vi "Progress Bar Example with Multiple Instances.vi"() -> ()   [LabVIEW 2015]
uses:
  Library/New Job Status.vi
  Library/New Item Status.vi
  Library/Class/Finish.vi
  Library/Class/Bar.lvclass
  Library/Simple Progress Bar.lvlib
panel:
  out "Action in Progress 2":bool=TRUE
  out "Action in Progress":bool=TRUE
  out "error out 2":errorcluster
  in  "Step Duration mSec 2":u32=100
  in  "Steps 2":i32=150
  in  "Step Duration mSec":u32=1000
  in  "Steps":i32=10
  out "error out":errorcluster
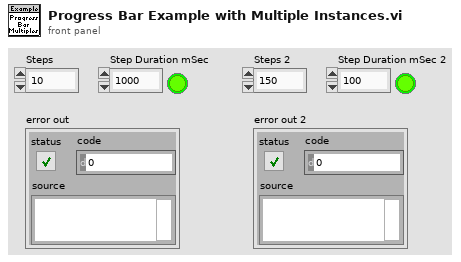
[diagram p1: front panel]
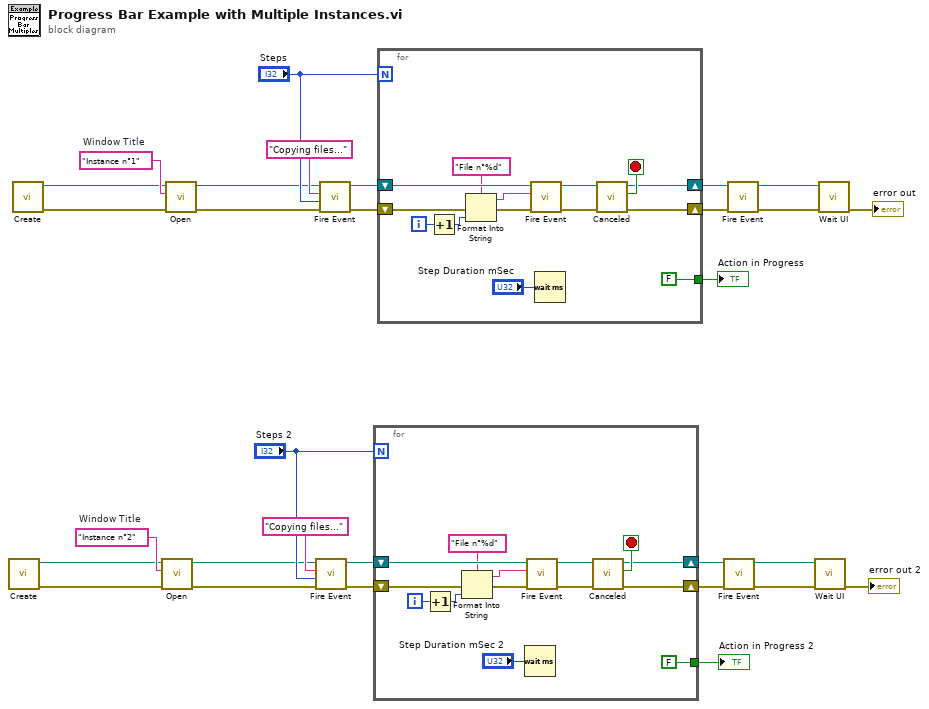
[diagram p0: block diagram]
diagram:
  w9 = "Instance n°2"  # Window Title
  w29 = "Instance n°1"  # Window Title
  n1 = call "Create.vi"() -> ("error out"=w8:errorcluster, "Bar out"=w5:refnum<class "Bar.lvclass">)  [unwired: 10 in]
  n2 = call "Create.vi"() -> ("error out"=w30:errorcluster, "Bar out"=w6:refnum<class "Bar.lvclass">)  [unwired: 10 in]
  n3 = call "Open.vi"("error in (no error)"=w8, "Window Title"=w9, "Bar in"=w5) -> ("error out"=w10:errorcluster, "Bar out"=w3:refnum<class "Bar.lvclass">)  [unwired: 7 in]
  n4 = call "Open.vi"("error in (no error)"=w30, "Window Title"=w29, "Bar in"=w6) -> ("error out"=w28:errorcluster, "Bar out"=w4:refnum<class "Bar.lvclass">)  [unwired: 7 in]
  n5 = call-poly "Fire Event.vi"("error in (no error)"=w10, "Items (unknown)"="Steps 2", "Status"="Copying files...", "Bar in"=w3) -> ("error out"=w12:errorcluster, "Bar out"=w11:refnum<class "Bar.lvclass">)  [unwired: 6 in]
  n6 = call-poly "Fire Event.vi"("error in (no error)"=w28, "Items (unknown)"="Steps", "Status"="Copying files...", "Bar in"=w4) -> ("error out"=w26:errorcluster, "Bar out"=w27:refnum<class "Bar.lvclass">)  [unwired: 6 in]
  n7 = for {
    N: "Steps 2" -> [_]
    shift-right: [w39] -> w18
    shift-left: w12 -> [w44]
    shift-right: [w31] -> w17
    shift-left: w11 -> [w42]
    tunnel: [FALSE] -> w7
    i -> [w41]
    stop <- w38 stop-if-true
    n8 = Increment(x=w41) -> (x+1=w34:i32)
    n9 = Format Into String(format string="File n°%d", error in=w44, w34) -> (resulting string=w35:string, error out=w36:errorcluster)  [unwired: 1 in]
    n10 = Wait (ms)(milliseconds to wait="Step Duration mSec 2") -> ()  [unwired: 1 out]
    n11 = call-poly "Fire Event.vi"("error in (no error)"=w36, "Status"=w35, "Bar in"=w42) -> ("error out"=w40:errorcluster, "Bar out"=w32:refnum<class "Bar.lvclass">)  [unwired: 7 in]
    n12 = call "Canceled.vi"("error in (no error)"=w40, "Bar in"=w32) -> ("error out"=w39:errorcluster, "Canceled by user?"=w38:bool, "Bar out"=w31:refnum<class "Bar.lvclass">)  [unwired: 7 in]
  }
  "Action in Progress 2" <- w7
  n13 = for {
    N: "Steps" -> [_]
    shift-right: [w53] -> w20
    shift-left: w26 -> [w58]
    shift-right: [w45] -> w21
    shift-left: w27 -> [w56]
    tunnel: [FALSE] -> w19
    i -> [w55]
    stop <- w52 stop-if-true
    n14 = Increment(x=w55) -> (x+1=w48:i32)
    n15 = Format Into String(format string="File n°%d", error in=w58, w48) -> (resulting string=w49:string, error out=w50:errorcluster)  [unwired: 1 in]
    n16 = call-poly "Fire Event.vi"("error in (no error)"=w50, "Status"=w49, "Bar in"=w56) -> ("error out"=w54:errorcluster, "Bar out"=w46:refnum<class "Bar.lvclass">)  [unwired: 7 in]
    n17 = Wait (ms)(milliseconds to wait="Step Duration mSec") -> ()  [unwired: 1 out]
    n18 = call "Canceled.vi"("error in (no error)"=w54, "Bar in"=w46) -> ("error out"=w53:errorcluster, "Canceled by user?"=w52:bool, "Bar out"=w45:refnum<class "Bar.lvclass">)  [unwired: 7 in]
  }
  "Action in Progress" <- w19
  n19 = call-poly "Fire Event.vi"("error in (no error)"=w18, "Bar in"=w17) -> ("error out"=w15:errorcluster, "Bar out"=w2:refnum<class "Bar.lvclass">)  [unwired: 8 in]
  n20 = call-poly "Fire Event.vi"("error in (no error)"=w20, "Bar in"=w21) -> ("error out"=w23:errorcluster, "Bar out"=w1:refnum<class "Bar.lvclass">)  [unwired: 8 in]
  n21 = call "Wait UI.vi"("error in (no error)"=w15, "Bar in"=w2) -> ("error out"=→"error out 2":errorcluster)  [unwired: 6 in, 3 out]
  n22 = call "Wait UI.vi"("error in (no error)"=w23, "Bar in"=w1) -> ("error out"=→"error out":errorcluster)  [unwired: 6 in, 3 out]
